vi "Create IMAQ Refs.vi"(8 "error in (no error)":errorcluster) -> (0 "error out":errorcluster, 4 "IMAQ Refs Dani":T1)   [LabVIEW 2015]
uses:
  TypeDefs Host/IMAQ Refs.ctl
  <vilib>/vision/Image Controls.llb/IMAQ Image.ctl
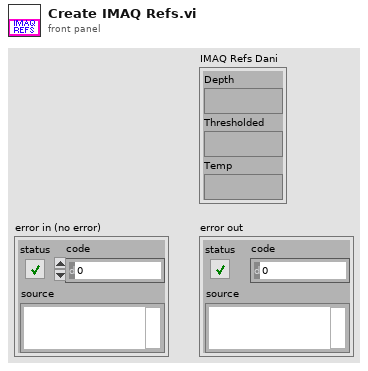
[diagram p1: front panel]
types:
  T1 = typedef "IMAQ Refs.ctl" = cluster{"Thresholded":T2, "Temp":T2, "Depth":T2}
  T2 = typedef "IMAQ Image.ctl" = refnum<image>
  T3 = typedef "Image Type" = u32
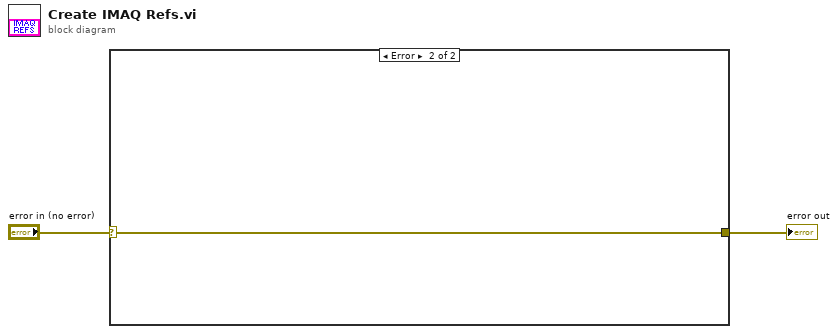
[diagram p0: block diagram]
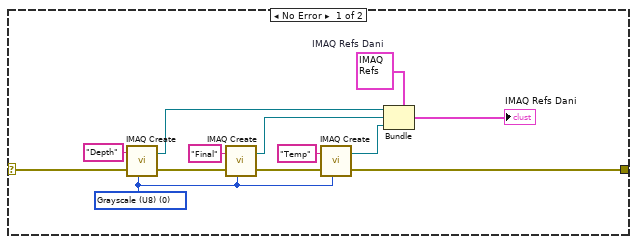
[diagram p2: hidden frame]
diagram:
  n1 = case shown="Error" "error in (no error)" {
    selector: "error in (no error)" -> [w3 w16]
    tunnel: [w15 w16] -> w2
    frame No Error {
      w4 = T1 {"Thresholded"=refnum, "Temp"=refnum, "Depth"=refnum}  # IMAQ Refs Dani
      w13 = T3 0 items=["Grayscale (U8)", "Grayscale (I16)", "Grayscale (SGL)", "Complex (CSG)", "RGB (U32)", "HSL (U32)", "RGB (U64)", "Grayscale (U16)"] ("Image Type")
      n2 = call "IMAQ Create"("Image Name"="Depth", "Image Type"=w13, "error in (no error)"=w3) -> ("New Image"=w12:T2, "error out"=w8:errorcluster)  [unwired: 2 in]
      n3 = call "IMAQ Create"("Image Name"="Final", "Image Type"=w13, "error in (no error)"=w8) -> ("New Image"=w11:T2, "error out"=w9:errorcluster)  [unwired: 2 in]
      n4 = call "IMAQ Create"("Image Name"="Temp", "Image Type"=w13, "error in (no error)"=w9) -> ("New Image"=w10:T2, "error out"=w15:errorcluster)  [unwired: 2 in]
      n5 = Bundle(cluster=w4, "Thresholded"=w12, "Temp"=w11, "Depth"=w10) -> (→"IMAQ Refs Dani":T1)
    }
    frame Error {
    }
  }
  "error out" <- w2
